vi "problem1.vi"() -> ()   [LabVIEW 2017]
panel:
  out "X2":dbl
  out "Area / X1":dbl
  in  "Cluster":T1
  in  "stop":bool
  in  "Enum":T2(ring)
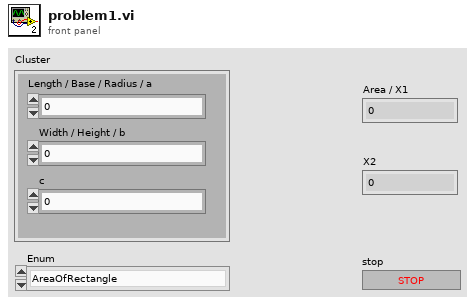
[diagram p1: front panel]
types:
  T1 = cluster{"Length / Base / Radius / a":dbl, "Width / Height / b":dbl, "c":dbl}
  T2 = enum16{"AreaOfRectangle", "AreaOfTriangle", "AreaOfCircle", "QuadraticEquation", "SquareRootOfPositiveNumber", ""}
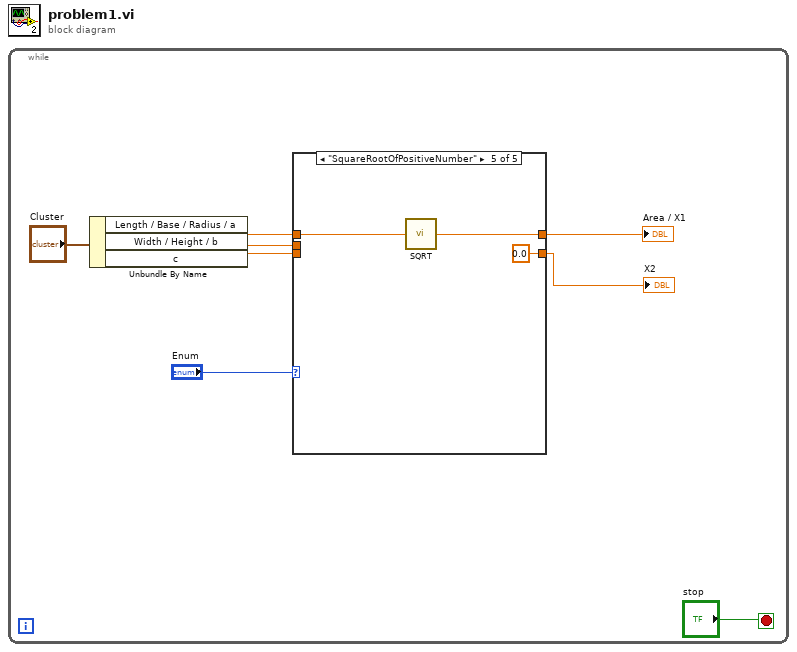
[diagram p0: block diagram]
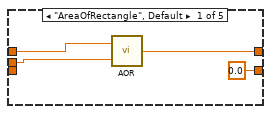
[diagram p2: hidden frame]
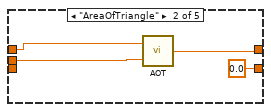
[diagram p3: hidden frame]
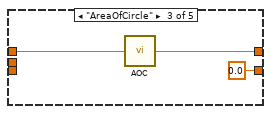
[diagram p4: hidden frame]
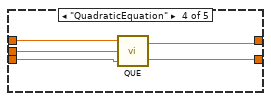
[diagram p5: hidden frame]
diagram:
  n1 = while {
    stop <- "stop" stop-if-true
    n2 = Unbundle By Name("Cluster") -> ("Length / Base / Radius / a"=w5:dbl, "Width / Height / b"=w4:dbl, "c"=w3:dbl)
    n3 = case shown="\"SquareRootOfPositiveNumber\"" "Enum" {
      tunnel: w5 -> [w12 w16 w19 w23 w27]
      tunnel: w4 -> [w11 w15 _ w22 _]
      tunnel: [w10 w14 w18 w24 w26] -> w2
      tunnel: w3 -> [_ _ _ w21 _]
      tunnel: [0.0 ("x2") 0.0 ("x2") 0.0 ("x2") w20 0.0 ("x2")] -> w1
      frame "AreaOfRectangle", Default {
        n4 = call "AOR.vi"("Length"=w11, "Width"=w12) -> ("Output"=w10:dbl)
      }
      frame "AreaOfTriangle" {
        n5 = call "AOT.vi"("height"=w15, "base"=w16) -> ("output"=w14:dbl)
      }
      frame "AreaOfCircle" {
        n6 = call "AOC.vi"("radius"=w19) -> ("output"=w18:dbl)
      }
      frame "QuadraticEquation" {
        n7 = call "QUE.vi"("C"=w21, "B"=w22, "A"=w23) -> ("x2"=w20:dbl, "x1"=w24:dbl)
      }
      frame "SquareRootOfPositiveNumber" {
        n8 = call "SQRT.vi"("Number"=w27) -> ("Square Root"=w26:dbl)
      }
    }
    "Area / X1" <- w2
    "X2" <- w1
  }
